vi "Get Authorization.vi"() -> (0 "error out":errorcluster, 3 "escaped string out":string)   [LabVIEW 2019]
uses:
  <vilib>/wsapi/NI_WebServices.lvlib
panel:
  in  "error in (no error)":errorcluster
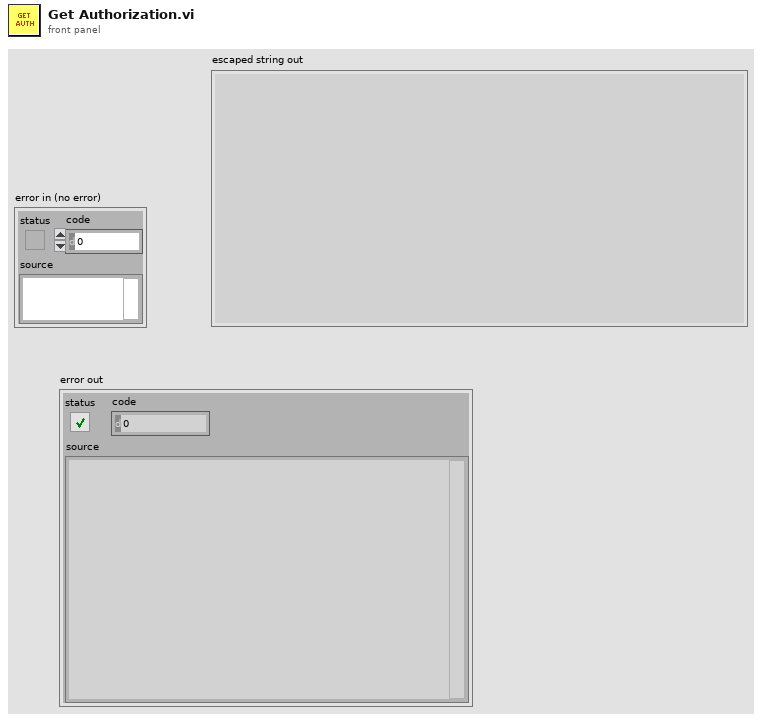
[diagram p1: front panel]
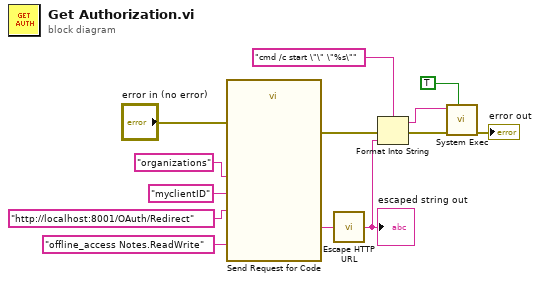
[diagram p0: block diagram]
diagram:
  n1 = call "Send Request for Code"("scopes"="offline_access Notes.ReadWrite", "tenant"="organizations", "clientID"="myclientID", "redirectURI"="http://localhost:8001/OAuth/Redirect", "error in (no error)"="error in (no error)") -> ("Result"=w12:string, "error out"=w3:errorcluster)  [unwired: 9 in]
  n2 = call <vilib>:"Escape HTTP URL.vi"("unescaped string in"=w12) -> ("escaped string out"=w8:string)
  "escaped string out" <- w8
  n3 = Format Into String(format string="cmd /c start \"\" \"%s\"" ("command line"), error in=w3, w8) -> (resulting string=w10:string, error out=w2:errorcluster)  [unwired: 1 in]
  n4 = call <vilib>:"System Exec.vi"("wait until completion? (T)"=TRUE, "error in (no error)"=w2, "command line"=w10) -> ("error out"=→"error out":errorcluster)  [unwired: 5 in, 3 out]
